vi "Parallel Loop Control Using Local Variable.vi"() -> ()   [LabVIEW 2016]
panel:
  out "Count 2":dbl
  in  "STOP":bool
  out "Count 1":dbl
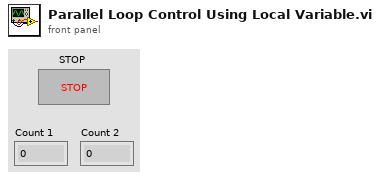
[diagram p1: front panel]
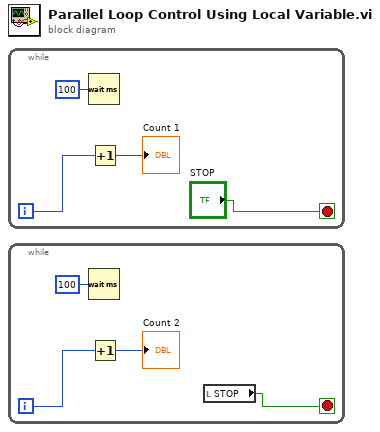
[diagram p0: block diagram]
diagram:
  n1 = while {
    i -> [w4]
    stop <- "STOP" stop-if-true
    n2 = Wait (ms)(milliseconds to wait=u32 100) -> ()  [unwired: 1 out]
    n3 = Increment(x=w4) -> (x+1=→"Count 1":i32)
  }
  n4 = while {
    i -> [w8]
    stop <- w5 stop-if-true
    n5 = Wait (ms)(milliseconds to wait=u32 100) -> ()  [unwired: 1 out]
    n6 = Increment(x=w8) -> (x+1=→"Count 2":i32)
    n7 = local read "STOP"() -> (w5:bool)
  }
